vi "Send due messages.vi"(10 "Scheduled messages in":T1[](array[typedef]), 11 "RT Queues":T2) -> (3 "Scheduled messages out":T1[](array[typedef]))   [LabVIEW 2018, in "Message scheduler.lvlib"]
uses:
  Message Scheduler/Message scheduler.lvlib
  Type Defs/Queues cluster.ctl
  Chris VIs/Message Scheduler/message scheduler.lvclass
  Type Defs/scheduled message cluster.ctl
types:
  T1 = typedef "Message scheduler.lvlib/scheduled message cluster.ctl" = cluster{"message element":cluster{"Message":string, "Data":variant}, "schedule":cluster{"Repeats":i16, "Period (ms)":u32, "ID":u32, "Queue":enum16{"Message", "Comms"}, "T0":u32}, "Action":enum16{"New", "Remove", "Quit"}}
  T2 = typedef "Queues cluster.ctl" = cluster{"RT Message":refnum<queue>, "RT Comms":refnum<queue>, "RT Data":refnum<queue>, "RT FIFO":refnum<queue>, "message scheduler":refnum<class "message scheduler.lvclass">}
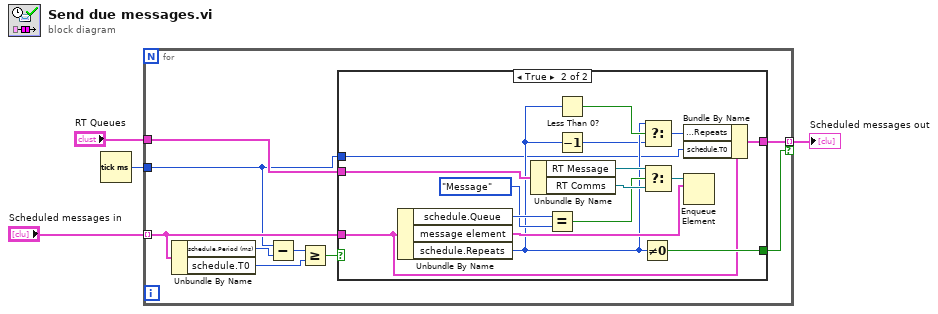
[diagram p0: block diagram]
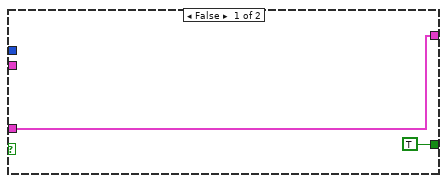
[diagram p2: hidden frame]
diagram:
  n1 = Tick Count (ms)() -> (millisecond timer value=w1:u32)
  n2 = for {
    tunnel: [w8] -> w2 mode=indexing if=w6
    tunnel: "Scheduled messages in" -> [w9] mode=indexing
    tunnel: "RT Queues" -> [w10]
    tunnel: w1 -> [w5]
    n3 = Unbundle By Name(w9) -> ("schedule.Period (ms)"=w13:u32, "schedule.T0"=w11:u32)
    n4 = Subtract(x=w5, y=w13) -> (x-y=w12:u32)
    n5 = Greater Or Equal?(x=w12, y=w11) -> (x >= y?=w7:bool)
    n6 = case shown="True" w7 {
      tunnel: w10 -> [_ w31]
      tunnel: w9 -> [w15 w22]
      tunnel: [w15 w21] -> w8
      tunnel: [TRUE w23] -> w6
      tunnel: w5 -> [_ w16]
      frame False {
      }
      frame True {
        n7 = Unbundle By Name(w22) -> ("schedule.Queue"=w28:enum16{"Message", "Comms"}, "message element"=w24:cluster{"Message":string, "Data":variant}, "schedule.Repeats"=w18:i16)
        n8 = Unbundle By Name(w31) -> ("RT Message"=w30:refnum<queue>, "RT Comms"=w29:refnum<queue>)
        n9 = Equal?(x=w28, y=enum16{"Message", "Comms"}."Message" ("schedule.Queue")) -> (x = y?=w26:bool)
        n10 = Less Than 0?(x=w18) -> (x < 0?=w20:bool)
        n11 = Decrement(x=w18) -> (x-1=w17:i16)
        n12 = Not Equal To 0?(x=w18) -> (x != 0?=w23:bool)
        n13 = Select(t=w18, s=w20, f=w17) -> (s? t:f=w19:i16)
        n14 = Select(t=w30, s=w26, f=w29) -> (s? t:f=w25:refnum<queue>)
        n15 = Bundle By Name(cluster=w22, "schedule.Repeats"=w19, "schedule.T0"=w16) -> (w21:T1)
        n16 = Enqueue Element(queue=w25, element=w24) -> ()  [unwired: 2 in, 3 out]
      }
    }
  }
  "Scheduled messages out" <- w2
